vi "Queue.vi"(8 "error in":errorcluster, 9 "Message Data":variant, 10 "Message":string, 11 "Function":T2(ring)) -> (0 "error out":errorcluster, 2 "Release Queue":T1[](array[typedef]), 3 "queue out":refnum<queue>)   [LabVIEW 2016]
uses:
  Message Queue/Message Cluster.ctl
  Message Queue/Message Queue.lvlib
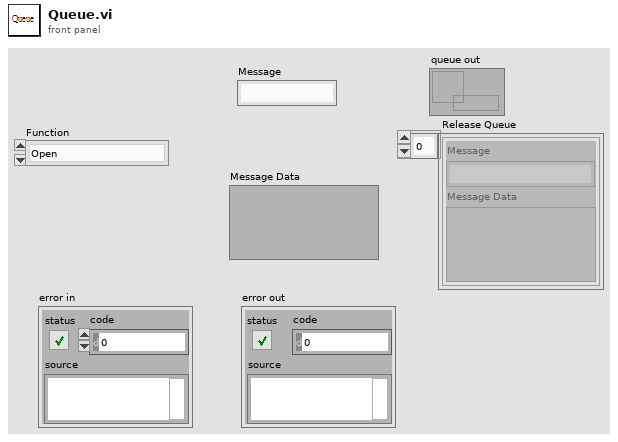
[diagram p1: front panel]
types:
  T1 = typedef "Message Queue.lvlib/Message Cluster.ctl" = cluster{"Message":string, "Message Data":variant}
  T2 = enum16{"Open", "Enqueue", "InsertQueue", "Release Queue", "Close"}
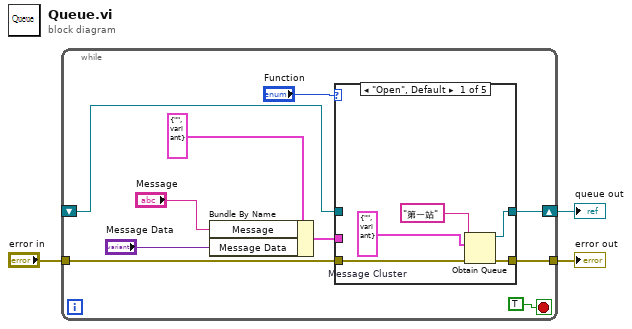
[diagram p0: block diagram]
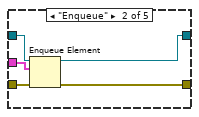
[diagram p2: hidden frame]
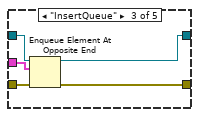
[diagram p3: hidden frame]
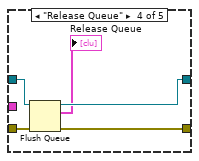
[diagram p4: hidden frame]
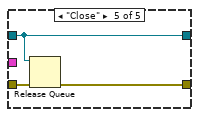
[diagram p5: hidden frame]
diagram:
  n1 = while {
    shift-right: [w11] -> w1
    shift-left: _ -> [w10]
    tunnel: "error in" -> [w9]
    tunnel: [w8] -> w2
    stop <- TRUE stop-if-true
    n2 = Bundle By Name(cluster=T1 {"Message"="", "Message Data"=variant} ("element 2"), "Message"="Message", "Message Data"="Message Data") -> (w4:T1)
    n3 = case shown="\"Open\", Default" "Function" {
      tunnel: [w18 w23 w27 w32 w36] -> w11
      tunnel: w10 -> [_ w22 w28 w33 w36]
      tunnel: w9 -> [w17 w20 w25 w30 w35]
      tunnel: [w16 w21 w26 w31 w34] -> w8
      tunnel: w4 -> [_ w19 w24 _ _]
      frame "Open", Default {
        w15 = T1 {"Message"="", "Message Data"=variant}  # Message Cluster
        n4 = Obtain Queue(name (unnamed)="第一站", element data type=w15, error in (no error)=w17) -> (queue out=w18:refnum<queue>, error out=w16:errorcluster)  [unwired: 2 in, 1 out]
      }
      frame "Enqueue" {
        n5 = Enqueue Element(queue=w22, element=w19, error in (no error)=w20) -> (queue out=w23:refnum<queue>, error out=w21:errorcluster)  [unwired: 1 in, 1 out]
      }
      frame "InsertQueue" {
        n6 = Enqueue Element At Opposite End(queue=w28, element=w24, error in (no error)=w25) -> (queue out=w27:refnum<queue>, error out=w26:errorcluster)  [unwired: 1 in, 1 out]
      }
      frame "Release Queue" {
        n7 = Flush Queue(queue=w33, error in (no error)=w30) -> (queue out=w32:refnum<queue>, remaining elements=→"Release Queue":T1[], error out=w31:errorcluster)
      }
      frame "Close" {
        n8 = Release Queue(queue=w36, error in (no error)=w35) -> (error out=w34:errorcluster)  [unwired: 1 in, 2 out]
      }
    }
  }
  "error out" <- w2
  "queue out" <- w1
